vi "Check Time.vi"(8 "error in (no error)":errorcluster, 11 "Integrator in":refnum<class "Integrator.lvclass">) -> (0 "error out":errorcluster, 2 "Integrating":bool, 3 "Integrator out":refnum<class "Integrator.lvclass">)   [LabVIEW 2016, in "Integrator.lvclass"]
uses:
  Integrator.lvclass
  Integrator.lvclass/Integrator.ctl
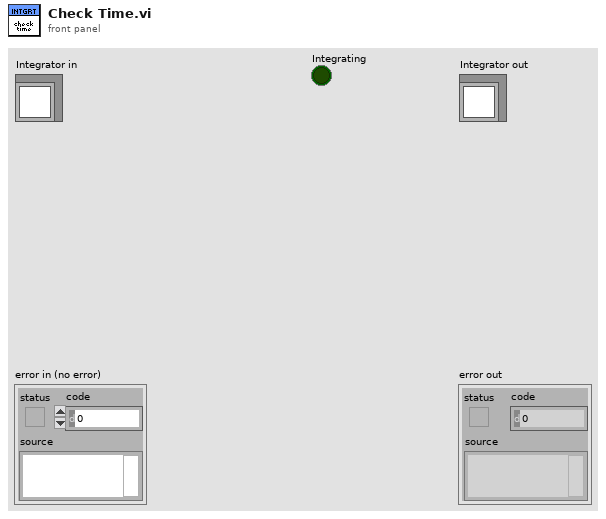
[diagram p1: front panel]
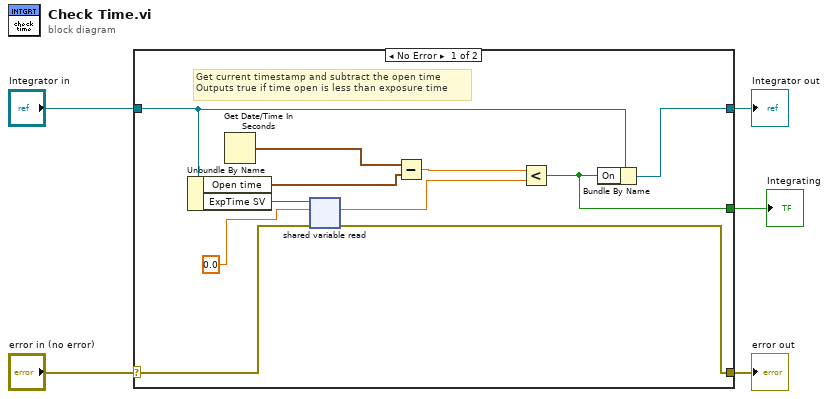
[diagram p0: block diagram]
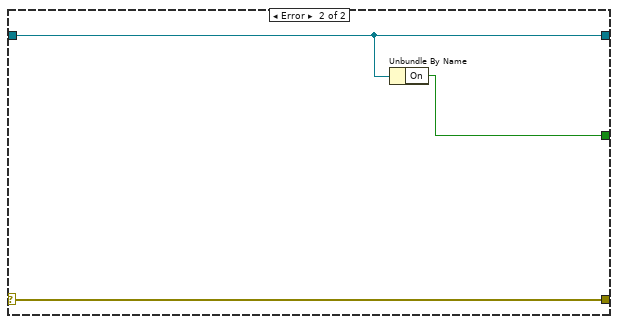
[diagram p2: hidden frame]
diagram:
  n1 = case shown="No Error" "error in (no error)" {
    selector: "error in (no error)" -> [w10 w19]
    tunnel: [w9 w19] -> w4
    tunnel: [w12 w18] -> w2
    tunnel: "Integrator in" -> [w13 w18]
    tunnel: [w6 w17] -> w1
    frame No Error {
      # "Get current timestamp and subtract the open time\nOutputs true if time open is less than exposure time"
      n2 = Unbundle By Name(w13) -> ("Open time"=w15:timestamp, "ExpTime SV"=w11:refnum<k21>)
      n3 = Get Date/Time In Seconds() -> (seconds since 1Jan1904=w16:timestamp)
      n4 = shared-variable-read(w11, w10, 0.0) -> (w9:errorcluster, w7:dbl)  [unwired: 2 out]
      n5 = Subtract(x=w16, y=w15) -> (x-y=w14:dbl)
      n6 = Less?(x=w14, y=w7) -> (x < y?=w6:bool)
      n7 = Bundle By Name(cluster=w13, "On"=w6) -> (w12:refnum<class "Integrator.lvclass">)
    }
    frame Error {
      n8 = Unbundle By Name(w18) -> ("On"=w17:bool)
    }
  }
  "error out" <- w4
  "Integrator out" <- w2
  "Integrating" <- w1
